vi "rate safety.vi"(4 "Max Rate":dbl=50.0, 5 "Desired Rate":dbl, 6 "Cutoff Rate":dbl=0.2, 7 "Encoder Rate":dbl) -> (0 "Limit":bool, 1 "Cutoff Tripped":bool, 2 "Output Rate":dbl, 3 "Encoder Rate Out":dbl)   [LabVIEW 2013]
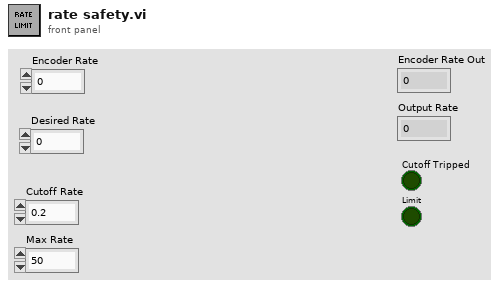
[diagram p1: front panel]
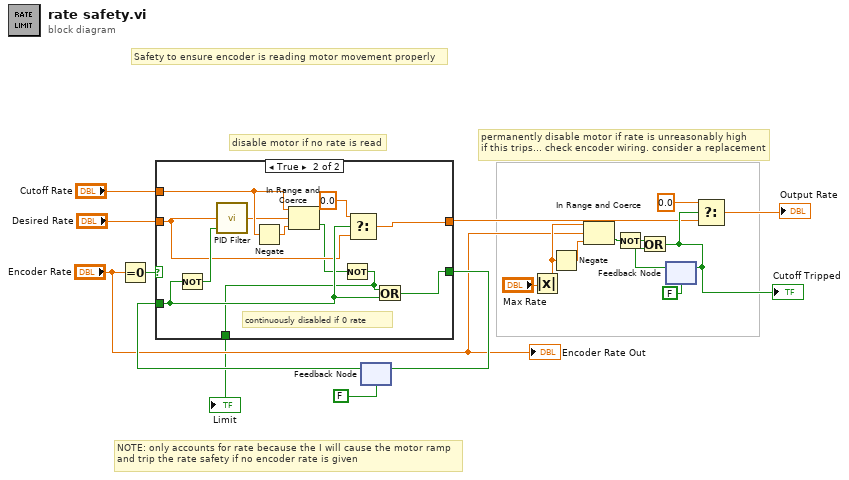
[diagram p0: block diagram]
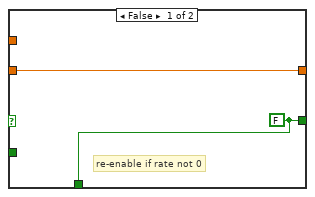
[diagram p2: hidden frame]
diagram:
  # "Safety to ensure encoder is reading motor movement properly"
  # "NOTE: only accounts for rate because the I will cause the motor ramp\nand trip the rate safety if no encoder rate is given"
  # "permanently disable motor if rate is unreasonably high\nif this trips... check encoder wiring. consider a replacement"
  # "disable motor if no rate is read"
  n1 = Equal To 0?(x="Encoder Rate") -> (x = 0?=w18:bool)
  n2 = feedback #1(FALSE ("x > y?")) -> (w11:bool)
  n3 = case shown="True" w18 {
    tunnel: "Desired Rate" -> [w21 w25]
    tunnel: [w21 w31] -> w8
    tunnel: [w20 w30] -> w6
    tunnel: w11 -> [_ w29]
    tunnel: "Cutoff Rate" -> [_ w27]
    tunnel: [w20 w22] -> w1
    frame False {
      w20 = FALSE
      # "re-enable if rate not 0"
    }
    frame True {
      # "continuously disabled if 0 rate"
      n4 = Not(x=w29) -> (.not. x?=w26:bool)
      n5 = call "PID Filter.vi"("reinitialize? (F)"=w26, "input"=w25) -> ("output"=w24:dbl)  [unwired: 3 in]
      n6 = Negate(x=w27) -> (-x=w28:dbl)
      n7 = In Range and Coerce(upper limit=w27, x=w24, lower limit=w28) -> (In Range?=w23:bool)  [unwired: 1 out]
      n8 = Not(x=w23) -> (.not. x?=w22:bool)
      n9 = Select(t=0.0, s=w29, f=w25) -> (s? t:f=w31:dbl)
      n10 = Or(x=w22, y=w29) -> (x .or. y?=w30:bool)
    }
  }
  "Limit" <- w1
  n11 = feedback-in #1(w6) -> ()
  n12 = Absolute Value(x="Max Rate") -> (abs(x)=w3:dbl)
  n13 = Negate(x=w3) -> (-x=w5:dbl)
  n14 = In Range and Coerce(upper limit=w3, x="Encoder Rate", lower limit=w5) -> (In Range?=w10:bool)  [unwired: 1 out]
  n15 = Not(x=w10) -> (.not. x?=w9:bool)
  n16 = feedback #2(FALSE ("x > y?")) -> (w15:bool)
  n17 = Or(x=w9, y=w15) -> (x .or. y?=w14:bool)
  "Cutoff Tripped" <- w14
  n18 = feedback-in #2(w14) -> ()
  n19 = Select(t=0.0, s=w14, f=w8) -> (s? t:f=→"Output Rate":dbl)
  "Encoder Rate Out" <- "Encoder Rate"
